vi "Init from Element.vi"(8 "error in (no error)":errorcluster, 10 "Config Element":refnum<class "Config Element.lvclass">, 11 "Transition Config in":refnum<class "Transition Config.lvclass">) -> (0 "error out":errorcluster, 3 "Transition Config out":refnum<class "Transition Config.lvclass">)   [LabVIEW 2020]
uses:
  Transition Config.lvclass
  lv-cdm/CDM-Config/Config Element/Config Element.lvclass
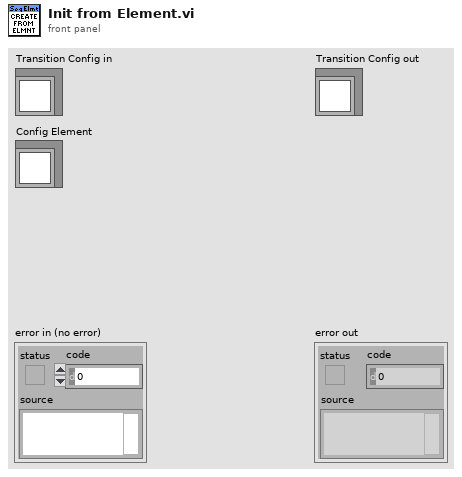
[diagram p1: front panel]
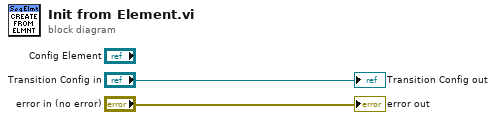
[diagram p0: block diagram]
diagram:
  "error out" <- "error in (no error)"
  "Transition Config out" <- "Transition Config in"
